vi "Set Current Camera.vi"(8 "error in (no error)":errorcluster, 11 "Channel in":refnum<class "Channel.lvclass">) -> (0 "error out":errorcluster, 3 "Channel out":refnum<class "Channel.lvclass">)   [LabVIEW 2018, in "Channel.lvclass"]
uses:
  Channel.lvclass
  Channel.lvclass/Channel.ctl
  Simulated_CCD_Camera/Simulated_CCD_Camera.lvclass
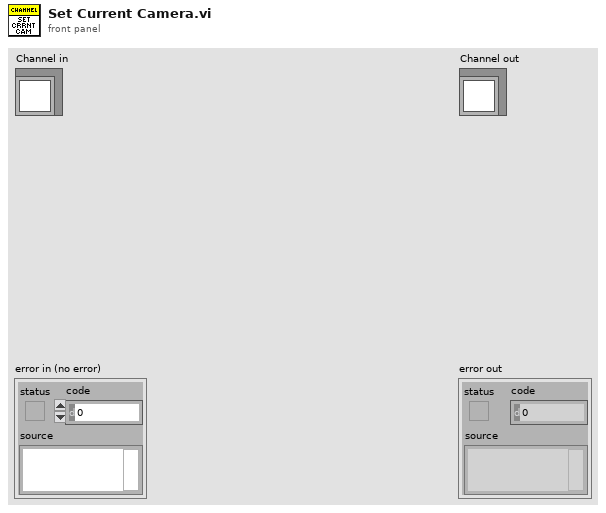
[diagram p1: front panel]
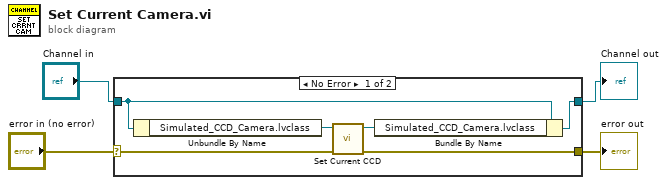
[diagram p0: block diagram]
diagram:
  n1 = case shown="No Error" "error in (no error)" {
    selector: "error in (no error)" -> [w5 w12]
    tunnel: [w7 w12] -> w3
    tunnel: [w9 w11] -> w1
    tunnel: "Channel in" -> [w10 w11]
    frame No Error {
      n2 = Unbundle By Name(w10) -> ("Simulated_CCD_Camera.lvclass"=w6:refnum<class "Simulated_CCD_Camera.lvclass">)
      n3 = call-dynamic "Set Current CCD.vi"("error in (no error)"=w5, "Simulated_CCD_Camera in"=w6) -> ("error out"=w7:errorcluster, "Simulated_CCD_Camera out"=w8:refnum<class "Simulated_CCD_Camera.lvclass">)  [unwired: 8 in]
      n4 = Bundle By Name(cluster=w10, "Simulated_CCD_Camera.lvclass"=w8) -> (w9:refnum<class "Channel.lvclass">)
    }
    frame Error {
    }
  }
  "error out" <- w3
  "Channel out" <- w1
